vi "Calculate_Wind_Chill.vi"(1 "Wind speed (mph)":sgl, 2 "Outside temperature (F)":sgl) -> (0 "Wind Chill (C)":sgl format="%#.1f")   [LabVIEW 2012]
panel:
  out "Wind Chill (F)":dbl
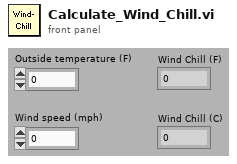
[diagram p1: front panel]
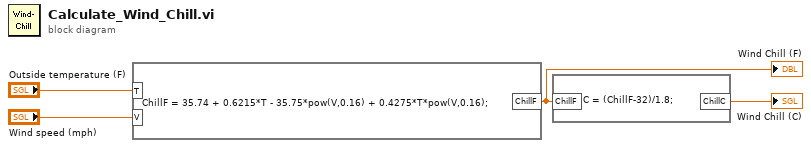
[diagram p0: block diagram]
diagram:
  n1 = formula code="ChillF = 35.74 + 0.6215*T - 35.75*pow(V,0.16) + 0.4275*T*pow(V,0.16);"("T"="Outside temperature (F)", "V"="Wind speed (mph)") -> ("ChillF"=w1:dbl)
  "Wind Chill (F)" <- w1
  n2 = formula code="ChillC = (ChillF-32)/1.8;"("ChillF"=w1) -> ("ChillC"=→"Wind Chill (C)":dbl)
